vi "Error Query.vi"(8 "error in (no error)":errorcluster, 10 "parseError? (true)":bool=TRUE, 11 "VISA resource name":refnum<visa-resource-name>) -> (0 "error out":errorcluster, 1 "Code":i32, 2 "AnswerString (output)":string, 3 "VISA resource name out":refnum<visa-resource-name>)   [LabVIEW 2018, in "JULABO DeviceDriver.lvlib"]
doc: "Queries the instrument for any errors in the instrument's error queue. It will continue to read errors until all errors have been read from the instrument. Any errors will be returned in the Error Out cluster.\n\nNote:\nThis VI is called automatically by most driver VIs so it is not usually necessary to call this in an application."
uses:
  JULABO DeviceDriver.lvlib
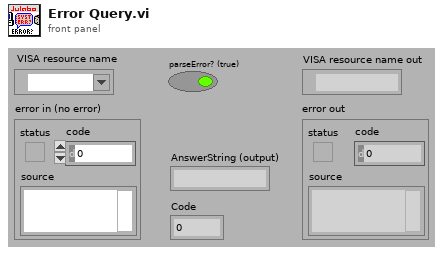
[diagram p1: front panel]
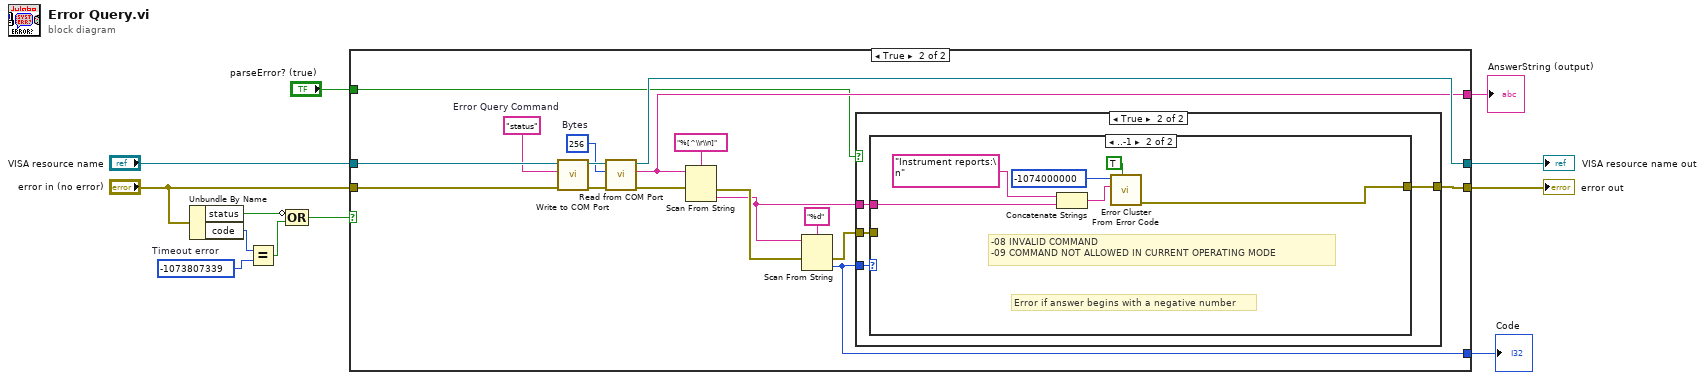
[diagram p0: block diagram]
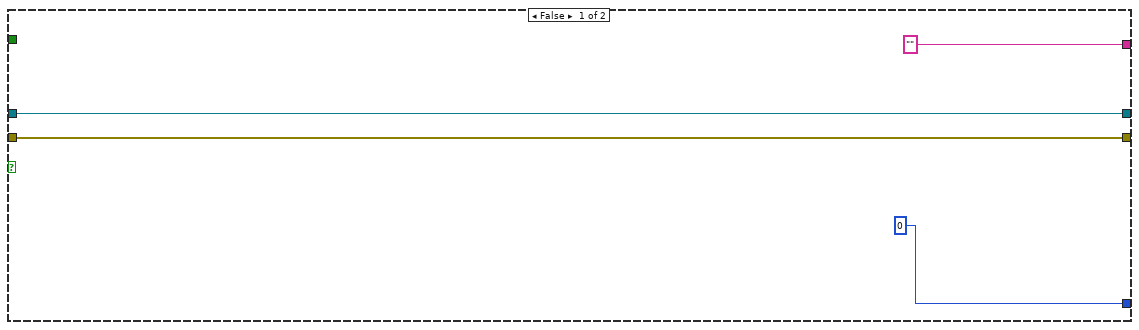
[diagram p2: hidden frame]
diagram:
  w5 = -1073807339  # Timeout error
  n1 = Unbundle By Name("error in (no error)") -> ("status"=w4:bool, "code"=w7:i32)
  n2 = Equal?(x=w7, y=w5) -> (x = y?=w6:bool)
  n3 = Compound Arithmetic op=OR(invert w4, w6) -> (w3:bool)
  n4 = case shown="True" w3 {
    tunnel: [w16 w22] -> w12
    tunnel: "VISA resource name" -> [w16 w33]
    tunnel: [w13 w24] -> w10
    tunnel: ["" ("String (output)") w21] -> w9
    tunnel: [0 w20] -> w8
    tunnel: "error in (no error)" -> [w13 w19]
    tunnel: "parseError? (true)" -> [_ w17]
    frame False {
    }
    frame True {
      w31 = u32 256  # Bytes
      w29 = "status"  # Error Query Command
      n5 = call "Write to COM Port.vi"("error in"=w19, "Command (input)"=w29, "VISA resource name in"=w33) -> ("error out"=w30:errorcluster, "VISA resource name out"=w32:refnum<visa-resource-name>)  [unwired: 7 in]
      n6 = call "Read from COM Port.vi"("error in"=w30, "Byte to Read (-1:All)"=w31, "VISA resource name in"=w32) -> ("error out"=w26:errorcluster, "String (output)"=w21:string, "VISA resource name out"=w22:refnum<visa-resource-name>)  [unwired: 5 in, 1 out]
      n7 = Scan From String(format string="%[^\\r\\n]", input string=w21, error in=w26) -> (error out=w25:errorcluster, output 1=w18:string)  [unwired: 2 in, 2 out]
      n8 = Scan From String(format string="%d", input string=w18, error in=w25) -> (error out=w23:errorcluster, output 1=w20:i32)  [unwired: 2 in, 2 out]
      n9 = case shown="True" w17 {
        tunnel: w20 -> [_ w38]
        tunnel: w18 -> [_ w37]
        tunnel: [w34 w36] -> w24
        tunnel: w23 -> [w34 w35]
        frame False {
        }
        frame True {
          n10 = case shown="..-1" w38 {
            tunnel: w37 -> [_ w41]
            tunnel: [w39 w40] -> w36
            tunnel: w35 -> [w39 _]
            frame Default {
            }
            frame ..-1 {
              # "Error if answer begins with a negative number"
              # "-08 INVALID COMMAND\n-09 COMMAND NOT ALLOWED IN CURRENT OPERATING MODE"
              n11 = Concatenate Strings("Instrument reports:\n" ("Source"), w41) -> (w45:string)
              n12 = call <vilib>:"Error Cluster From Error Code.vi"("show call chain? (False)"=TRUE, "error message (\"\")"=w45, "error code (0)"=-1074000000 ("Code")) -> ("error out"=w40:errorcluster)  [unwired: 6 in]
            }
          }
        }
      }
    }
  }
  "VISA resource name out" <- w12
  "error out" <- w10
  "AnswerString (output)" <- w9
  "Code" <- w8
